vi "CollectCorner (SubVI).vi"(0 "XYZ .NET Refnum in":refnum<k24>, 1 "Calibration [um/pix]":dbl, 2 "Placement tolerance [um]":dbl, 5 "Placement Monitor":T3, 7 "Fiducial Template":T3, 11 "error in (no error)":errorcluster, 12 "Axis Speeds":T1, 13 "Corner Coordinates":cluster{"X":dbl, "Y":dbl, "Z":dbl}) -> (4 "XYZ .NET Refnum out":refnum<k24>, 6 "Placement Monitor out":T3, 8 "Corner surveyed position":dbl[](array[numeric]), 10 "XYZ Stage Final Position":T2, 15 "error out":errorcluster)   [LabVIEW 2016]
uses:
  <vilib>/vision/Image Controls.llb/IMAQ Image.ctl
  C:/Users/Aerotech/Documents/BNLStaveAssembly-blueprint/Bin/Aerotech.A3200.dll
  BNLStaveAssembly-blueprint/Bin/Aerotech.A3200.dll
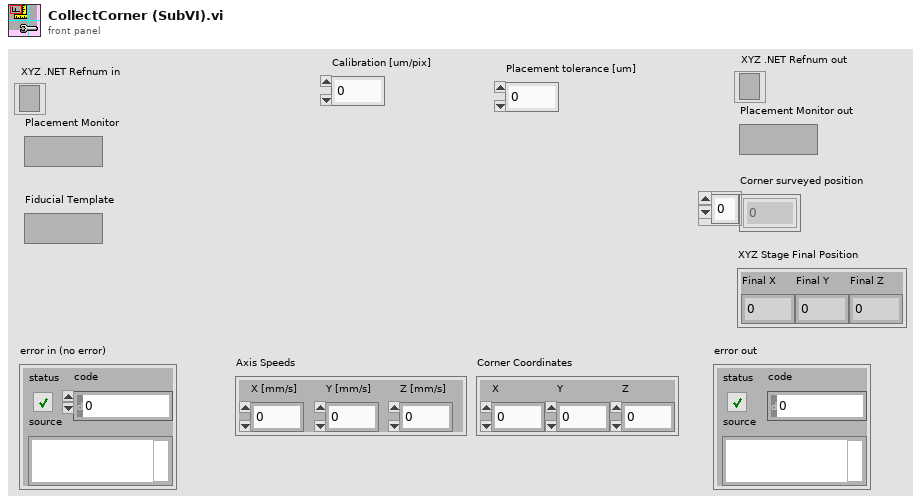
[diagram p1: front panel]
types:
  T1 = cluster{"X [mm/s]":dbl, "Y [mm/s]":dbl, "Z [mm/s]":dbl}
  T2 = cluster{"Final X":dbl, "Final Y":dbl, "Final Z":dbl}
  T3 = typedef "IMAQ Image.ctl" = refnum<image>
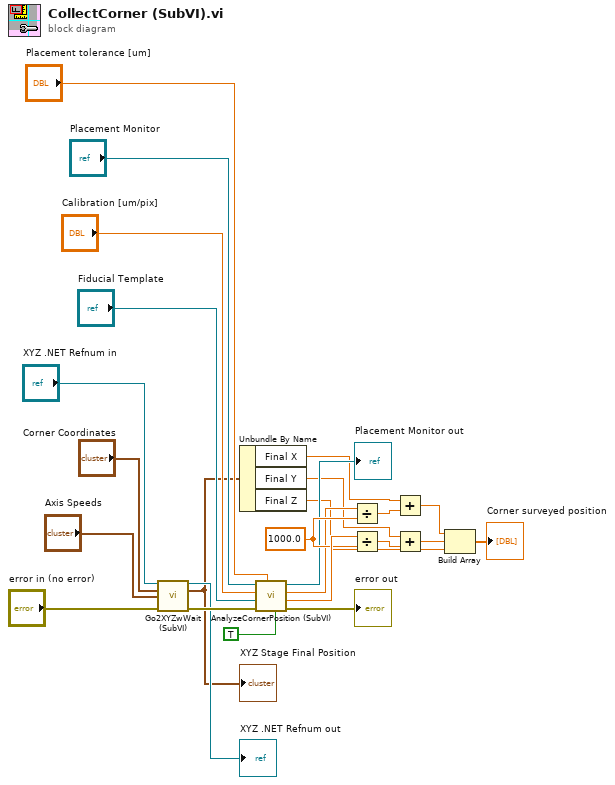
[diagram p0: block diagram]
diagram:
  w23 = sgl 1000.0 ("y")
  n1 = call "Go2XYZwWait (SubVI).vi"(".NET Refnum in"="XYZ .NET Refnum in", "Go to Coordinates"="Corner Coordinates", "Axis Speeds"="Axis Speeds", "error in (no error)"="error in (no error)") -> (".NET Refnum out"=→"XYZ .NET Refnum out":refnum<k24>, "Final Position"=w4:T2, "error out"=w18:errorcluster)  [unwired: 7 in, 2 out]
  "XYZ Stage Final Position" <- w4
  n2 = Unbundle By Name(w4) -> ("Final X"=w12:dbl, "Final Y"=w14:dbl, "Final Z"=w16:dbl)
  n3 = call "AnalyzeCornerPosition (SubVI).vi"("Center-only search?"=TRUE, "Placement tolerance [um]"="Placement tolerance [um]", "error in (no error)"=w18, "Fiducial Template"="Fiducial Template", "Calibration [um/pix]"="Calibration [um/pix]", "Refnum in"="Placement Monitor") -> ("error out"=→"error out":errorcluster, "Y offset [um]"=w24:sgl, "X offset [um]"=w21:sgl, "Refnum out"=→"Placement Monitor out":T3)  [unwired: 1 in, 1 out]
  n4 = Divide(x=w21, y=w23) -> (x/y=w22:sgl)
  n5 = Divide(x=w24, y=w23) -> (x/y=w25:sgl)
  n6 = Add(x=w12, y=w22) -> (x+y=w13:dbl)
  n7 = Add(x=w14, y=w25) -> (x+y=w15:dbl)
  n8 = Build Array(w13, w15, w16) -> (→"Corner surveyed position":dbl[])
